vi "Swerve Driveold.vi"(0 "X":dbl, 1 "Rot. Point X":dbl, 3 "Rot. Point Y":dbl, 5 "Y":dbl, 7 "Z":dbl, 11 "Error In":errorcluster, 12 "Robot Centric?":bool=TRUE, 13 "Autonomous?":bool, 14 "Yaw":dbl) -> (4 "Front Left Output":dbl, 6 "Front Right Output":dbl, 8 "Back Left Output":dbl, 10 "Back Right Output":dbl, 15 "Error Out":errorcluster)   [LabVIEW 2018]
uses:
  <vilib>/Rock Robotics/WPI/ThirdParty/Phoenix-LabVIEW/Motor Controller/Controls/CTRE_Phoenix_MotorControl_ControlMode.ctl
panel:
  in  "Robot Length":dbl=33.5
  in  "Robot Width":dbl=28.5
  # "Swerve Drive Teleoperated Control\nFRC Team 34"
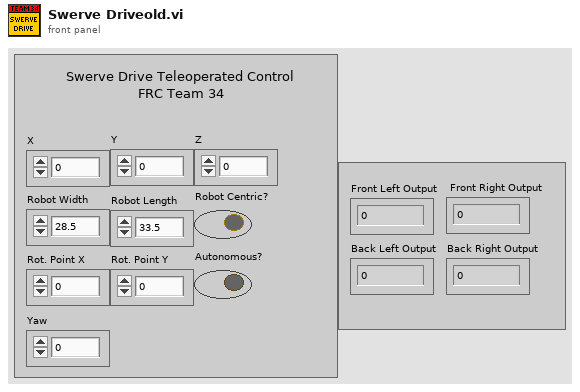
[diagram p1: front panel]
types:
  T1 = enum16{"Front Left", "Front Right", "Back Left", "Back Right"}
  T2 = typedef "CTRE_Phoenix_MotorControl_ControlMode.ctl" = u16
  T3 = typedef "WPI_MotorControlDeviceRef.ctl" = cluster{"DeviceStatus":errorcluster, "Type":T4, "PWM":cluster{"PWM Channel":T5, "DeadBand":T6}, "CAN":cluster{"Device Number":u8, "SetOutput VI Ref":variant, "GetOutput VI Ref":variant, "Enable VI Ref":variant, "Disable VI Ref":variant, "Data":variant}, "Invert":bool, "DIO PWM":cluster{"PWM \"Enable\" Channel":T5, "DIOChannel":T7, "PWM Rate":dbl}}
  T4 = typedef "WPI_MotorControlType.ctl" = enum16{"PWM", "CAN", "DIO PWM"}
  T5 = typedef "FPGA_DIOPWMChannel.ctl" = enum8{"PWM 0", "PWM 1", "PWM 2", "PWM 3", "PWM 4", "PWM 5", "PWM 6", "PWM 7", "PWM 8", "PWM 9", "PWM MXP 0", "PWM MXP 1", "PWM MXP 2", "PWM MXP 3", "PWM MXP 4", "PWM MXP 5", "PWM MXP 6", "PWM MXP 7", "PWM MXP 8", "PWM MXP 9", "Invalid"}
  T6 = typedef "WPI_PWMDeadband.ctl" = cluster{"Name":string, "maxPositivePwm":i32, "minPositivePwm":i32, "centerPwm":i32, "maxNegativePwm":i32, "minNegativePwm":i32, "angularRange":u16}
  T7 = typedef "FPGA_DIOChannel.ctl" = enum8{"DIO 0", "DIO 1", "DIO 2", "DIO 3", "DIO 4", "DIO 5", "DIO 6", "DIO 7", "DIO 8", "DIO 9", "DIO MXP 0", "DIO MXP 1", "DIO MXP 2", "DIO MXP 3", "DIO MXP 4", "DIO MXP 5", "DIO MXP 6", "DIO MXP 7", "DIO MXP 8", "DIO MXP 9", "DIO MXP 10", "DIO MXP 11", "DIO MXP 12", "DIO MXP 13", "DIO MXP 14", "DIO MXP 15", "SPI Port CS1", "SPI Port CS2", "SPI Port CS3", "SPI Port MISO", "SPI Port MOSI", "Invalid"}
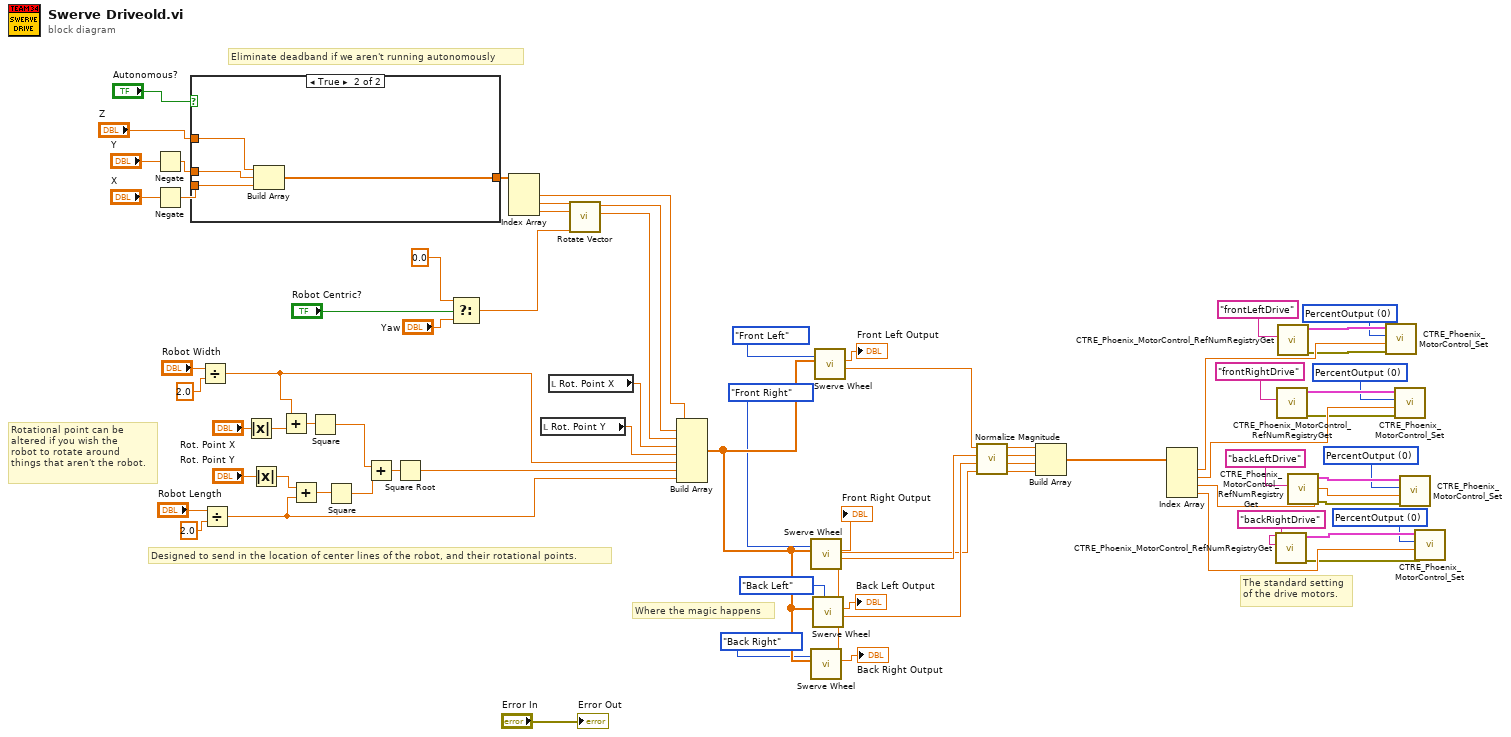
[diagram p0: block diagram]
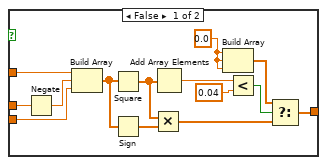
[diagram p2: hidden frame]
diagram:
  w7 = T2 0 items=["PercentOutput"=0, "Position"=1, "Velocity"=2, "Current"=3, "Follower"=5, "MotionProfile"=6, "MotionMagic"=7, "MotionMagicArc"=8, "MotionProfileArc"=10, "Disabled"=15] ("Control Mode")
  w8 = T2 0 items=["PercentOutput"=0, "Position"=1, "Velocity"=2, "Current"=3, "Follower"=5, "MotionProfile"=6, "MotionMagic"=7, "MotionMagicArc"=8, "MotionProfileArc"=10, "Disabled"=15] ("Control Mode")
  w9 = T2 0 items=["PercentOutput"=0, "Position"=1, "Velocity"=2, "Current"=3, "Follower"=5, "MotionProfile"=6, "MotionMagic"=7, "MotionMagicArc"=8, "MotionProfileArc"=10, "Disabled"=15] ("Control Mode")
  w10 = T2 0 items=["PercentOutput"=0, "Position"=1, "Velocity"=2, "Current"=3, "Follower"=5, "MotionProfile"=6, "MotionMagic"=7, "MotionMagicArc"=8, "MotionProfileArc"=10, "Disabled"=15] ("Control Mode")
  # "Rotational point can be \naltered if you wish the \nrobot to rotate around \nthings that aren't the robot."
  # "Eliminate deadband if we aren't running autonomously"
  # "Where the magic happens"
  # "The standard setting\nof the drive motors."
  # "Designed to send in the location of center lines of the robot, and their rotational points."
  n1 = Negate(x="Y") -> (-x=w28:dbl)
  n2 = Negate(x="X") -> (-x=w27:dbl)
  n3 = case shown="True" "Autonomous?" {
    tunnel: w28 -> [w77 w88]
    tunnel: [w76 w89] -> w72
    tunnel: "Z" -> [w75 w91]
    tunnel: w27 -> [w74 w90]
    frame False {
      w83 = 0.0 ("element")
      n4 = Negate(x=w77) -> (-x=w79:dbl)
      n5 = Build Array(w75, w79, w74) -> (w82:dbl[])
      n6 = Square(x=w82) -> (x^2=w80:dbl[])
      n7 = Sign(1:w82) -> (0:w81:dbl[])
      n8 = Multiply(x=w80, y=w81) -> (x*y=w78:dbl[])
      n9 = Add Array Elements(numeric array=w80) -> (sum=w87:dbl)
      n10 = Build Array(w83, w83, w83) -> (w84:dbl[])
      n11 = Less?(x=w87, y=0.04 ("x")) -> (x < y?=w85:bool)
      n12 = Select(t=w84, s=w85, f=w78) -> (s? t:f=w76:dbl[])
    }
    frame True {
      n13 = Build Array(w91, w88, w90) -> (w89:dbl[])
    }
  }
  n14 = Divide(x="Robot Width", y=2.0) -> (x/y=w46:dbl)
  n15 = Divide(x="Robot Length", y=2.0) -> (x/y=w44:dbl)
  n16 = Absolute Value(x="Rot. Point X") -> (abs(x)=w58:dbl)
  n17 = Absolute Value(x="Rot. Point Y") -> (abs(x)=w55:dbl)
  n18 = Add(x=w46, y=w58) -> (x+y=w57:dbl)
  n19 = Add(x=w55, y=w44) -> (x+y=w56:dbl)
  n20 = Square(x=w57) -> (x^2=w53:dbl)
  n21 = Square(x=w56) -> (x^2=w54:dbl)
  n22 = Add(x=w53, y=w54) -> (x+y=w52:dbl)
  n23 = Square Root(x=w52) -> (sqrt(x)=w45:dbl)
  n24 = Select(t=0.0, s="Robot Centric?", f="Yaw") -> (s? t:f=w65:dbl)
  n25 = Index Array(array=w72) -> (element #1=w51:dbl, element #2=w67:dbl, element #3=w66:dbl)  [unwired: 3 in]
  n26 = local read "Rot. Point Y"() -> (w47:dbl)
  n27 = local read "Rot. Point X"() -> (w48:dbl)
  n28 = call "Rotate Vector.vi"("Angle"=w65, "X"=w66, "Y"=w67) -> ("X'"=w49:dbl, "Y'"=w50:dbl)  [unwired: 7 in]
  n29 = Build Array(w51, w50, w49, w48, w47, w46, w45, w44) -> (w43:dbl[])
  n30 = call "Swerve Wheel.vi"("Wheel"=T1."Front Right", "Inputs"=w43) -> ("Speed"=w39:dbl, "Motor Output"=→"Front Right Output":dbl)  [unwired: 8 in]
  n31 = call "Swerve Wheel.vi"("Wheel"=T1."Back Right", "Inputs"=w43) -> ("Speed"=w37:dbl, "Motor Output"=→"Back Right Output":dbl)  [unwired: 8 in]
  n32 = call "Swerve Wheel.vi"("Wheel"=T1."Back Left", "Inputs"=w43) -> ("Speed"=w38:dbl, "Motor Output"=→"Back Left Output":dbl)  [unwired: 8 in]
  n33 = call "Swerve Wheel.vi"("Wheel"=T1."Front Left", "Inputs"=w43) -> ("Speed"=w40:dbl, "Motor Output"=→"Front Left Output":dbl)  [unwired: 8 in]
  n34 = call "Normalize Magnitude.vi"("D"=w37, "C"=w38, "B"=w39, "A"=w40) -> ("D'"=w33:dbl, "C'"=w34:dbl, "B'"=w35:dbl, "A'"=w36:dbl)  [unwired: 4 in]
  n35 = Build Array(w36, w35, w34, w33) -> (w1:dbl[])
  n36 = Index Array(array=w1) -> (element #1=w21:dbl, element #2=w15:dbl, element #3=w12:dbl, element #4=w18:dbl)  [unwired: 4 in]
  n37 = call <vilib>:"CTRE_Phoenix_MotorControl_RefNumRegistryGet.vi"("refnum name"="backRightDrive") -> ("error out"=w17:errorcluster, "PhoenixMotorControlDevRef"=w19:T3)  [unwired: 9 in]
  n38 = call <vilib>:"CTRE_Phoenix_MotorControl_RefNumRegistryGet.vi"("refnum name"="frontRightDrive") -> ("error out"=w14:errorcluster, "PhoenixMotorControlDevRef"=w16:T3)  [unwired: 9 in]
  n39 = call <vilib>:"CTRE_Phoenix_MotorControl_RefNumRegistryGet.vi"("refnum name"="frontLeftDrive") -> ("error out"=w20:errorcluster, "PhoenixMotorControlDevRef"=w22:T3)  [unwired: 9 in]
  n40 = call <vilib>:"CTRE_Phoenix_MotorControl_RefNumRegistryGet.vi"("refnum name"="backLeftDrive") -> ("error out"=w11:errorcluster, "PhoenixMotorControlDevRef"=w13:T3)  [unwired: 9 in]
  n41 = call <vilib>:"CTRE_Phoenix_MotorControl_Set.vi"("error in (no error)"=w20, "Output"=w21, "Control Mode"=w10, "PhoenixMotorControlDevRef"=w22) -> ()  [unwired: 6 in, 2 out]
  n42 = call <vilib>:"CTRE_Phoenix_MotorControl_Set.vi"("error in (no error)"=w14, "Output"=w15, "Control Mode"=w9, "PhoenixMotorControlDevRef"=w16) -> ()  [unwired: 6 in, 2 out]
  n43 = call <vilib>:"CTRE_Phoenix_MotorControl_Set.vi"("error in (no error)"=w11, "Output"=w12, "Control Mode"=w8, "PhoenixMotorControlDevRef"=w13) -> ()  [unwired: 6 in, 2 out]
  n44 = call <vilib>:"CTRE_Phoenix_MotorControl_Set.vi"("error in (no error)"=w17, "Output"=w18, "Control Mode"=w7, "PhoenixMotorControlDevRef"=w19) -> ()  [unwired: 6 in, 2 out]
  "Error Out" <- "Error In"
